vi "nonreentrant input.vi"(8 "error in (no error)":errorcluster, 10 "data table in in":T1, 11 "Queue in":refnum<queue>) -> (0 "error out":errorcluster, 3 "data table out":T1)   [LabVIEW 2013, in "testmod runtime.lvclass"]
uses:
  testmod runtime.lvclass
  <vilib>/NI/Tag Bus/table/data table.ctl
  <vilib>/NI/Tag Bus/table/data table.lvlib
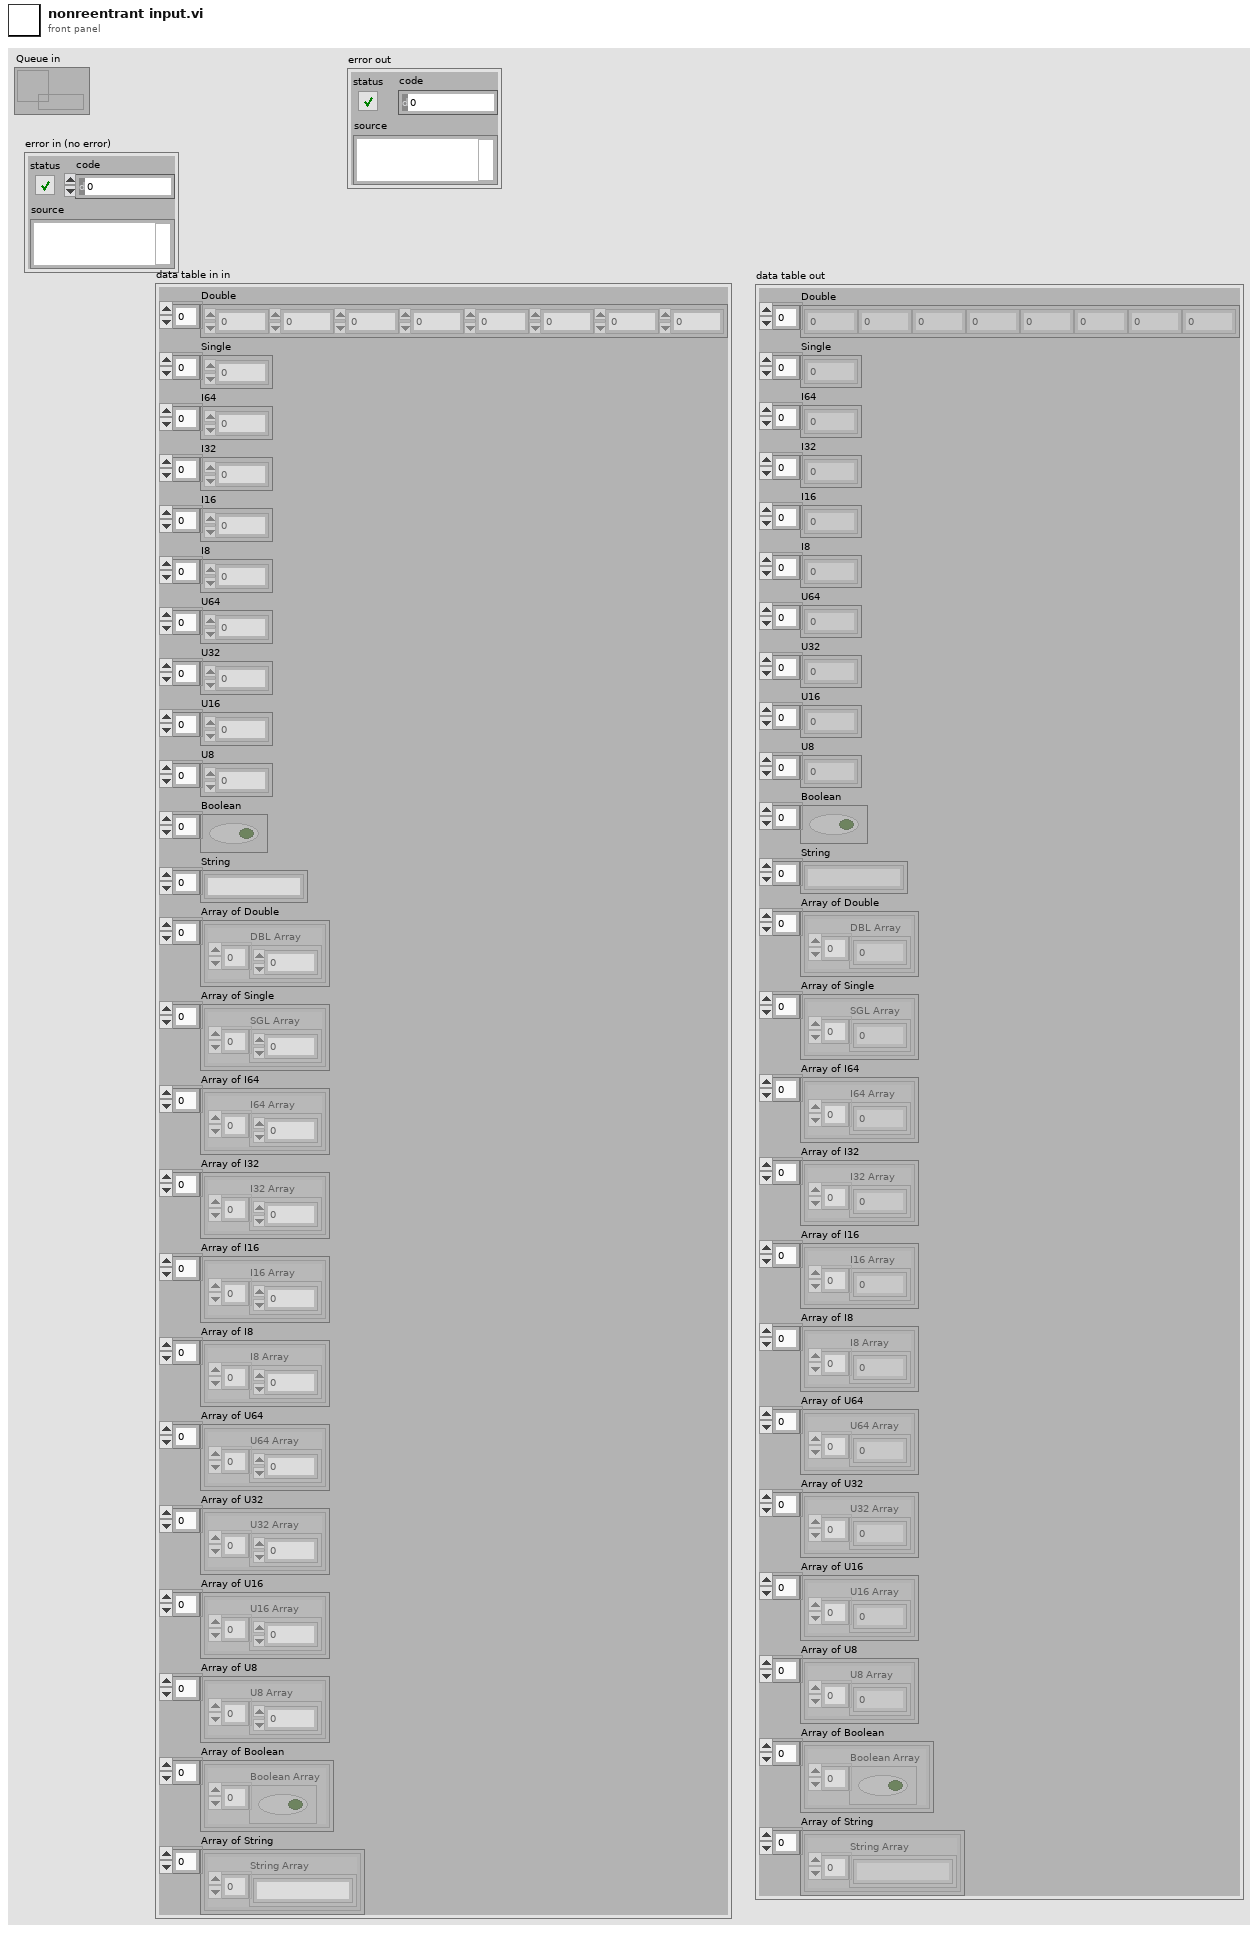
[diagram p1: front panel]
types:
  T1 = typedef "tag bus.lvlib/data table.lvlib/data table.ctl" = cluster{"Double":dbl[], "Single":sgl[], "I64":i64[], "I32":i32[], "I16":i16[], "I8":i8[], "U64":u64[], "U32":u32[], "U16":u16[], "U8":u8[], "Boolean":bool[], "String":string[], "Array of Double":cluster{"DBL Array":dbl[]}[], "Array of Single":cluster{"SGL Array":sgl[]}[], "Array of I64":cluster{"I64 Array":i64[]}[], "Array of I32":cluster{"I32 Array":i32[]}[], "Array of I16":cluster{"I16 Array":i16[]}[], "Array of I8":cluster{"I8 Array":i8[]}[], "Array of U64":cluster{"U64 Array":u64[]}[], "Array of U32":cluster{"U32 Array":u32[]}[], "Array of U16":cluster{"U16 Array":u16[]}[], "Array of U8":cluster{"U8 Array":u8[]}[], "Array of Boolean":cluster{"Boolean Array":bool[]}[], "Array of String":cluster{"String Array":string[]}[]}
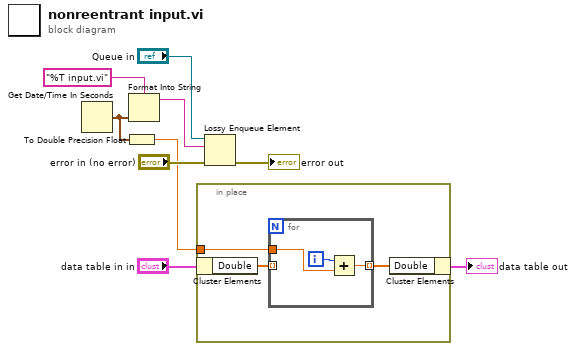
[diagram p0: block diagram]
diagram:
  n1 = Get Date/Time In Seconds() -> (seconds since 1Jan1904=w8:timestamp)
  n2 = To Double Precision Float(number=w8) -> (double precision float=w4:dbl)
  n3 = Format Into String(format string="%T input.vi", w8) -> (resulting string=w7:string)  [unwired: 2 in, 1 out]
  n4 = in-place {
    in-place-border: w4 -> [w11]
    n5 = in-place-cluster #1("data table in in") -> ("Double"=w12:dbl[])
    n6 = for {
      tunnel: w12 -> [_] mode=indexing
      tunnel: w11 -> [w14]
      tunnel: [w13] -> w10 mode=indexing
      i -> [w15]
      n7 = Add(x=w15, y=w14) -> (x+y=w13:dbl)
    }
    n8 = in-place-cluster #1("Double"=w10) -> (→"data table out":T1)
  }
  n9 = Lossy Enqueue Element(queue="Queue in", element=w7, error in (no error)="error in (no error)") -> (error out=→"error out":errorcluster)  [unwired: 3 out]
